vi "GetMotorStatus.vi"() -> (0 "status":T1)   [LabVIEW 2012]
panel:
  in  "簇":T1
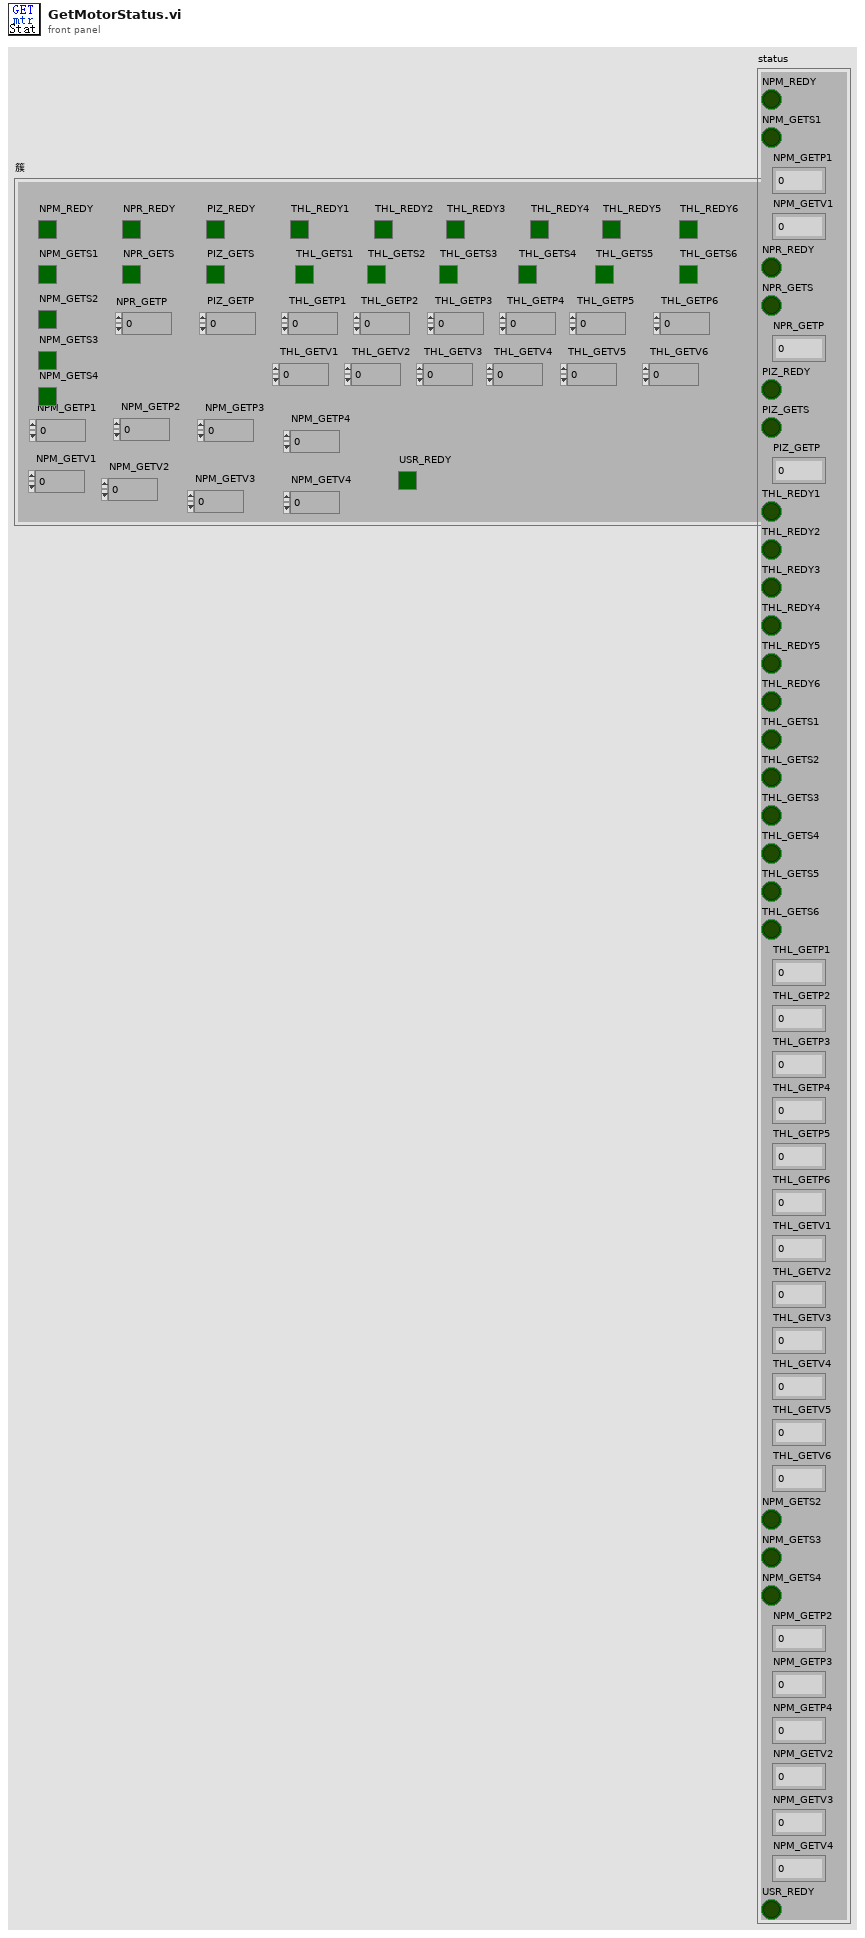
[diagram p1: front panel]
types:
  T1 = cluster{"NPM_REDY":bool, "NPM_GETS1":bool, "NPM_GETP1":dbl, "NPM_GETV1":dbl, "NPR_REDY":bool, "NPR_GETS":bool, "NPR_GETP":dbl, "PIZ_REDY":bool, "PIZ_GETS":bool, "PIZ_GETP":dbl, "THL_REDY1":bool, "THL_REDY2":bool, "THL_REDY3":bool, "THL_REDY4":bool, "THL_REDY5":bool, "THL_REDY6":bool, "THL_GETS1":bool, "THL_GETS2":bool, "THL_GETS3":bool, "THL_GETS4":bool, "THL_GETS5":bool, "THL_GETS6":bool, "THL_GETP1":dbl, "THL_GETP2":dbl, "THL_GETP3":dbl, "THL_GETP4":dbl, "THL_GETP5":dbl, "THL_GETP6":dbl, "THL_GETV1":dbl, "THL_GETV2":dbl, "THL_GETV3":dbl, "THL_GETV4":dbl, "THL_GETV5":dbl, "THL_GETV6":dbl, "NPM_GETS2":bool, "NPM_GETS3":bool, "NPM_GETS4":bool, "NPM_GETP2":dbl, "NPM_GETP3":dbl, "NPM_GETP4":dbl, "NPM_GETV2":dbl, "NPM_GETV3":dbl, "NPM_GETV4":dbl, "USR_REDY":bool}
  T2 = cluster{"DeviceID":string, "Channel":string, "param1":dbl, "Operation":string}
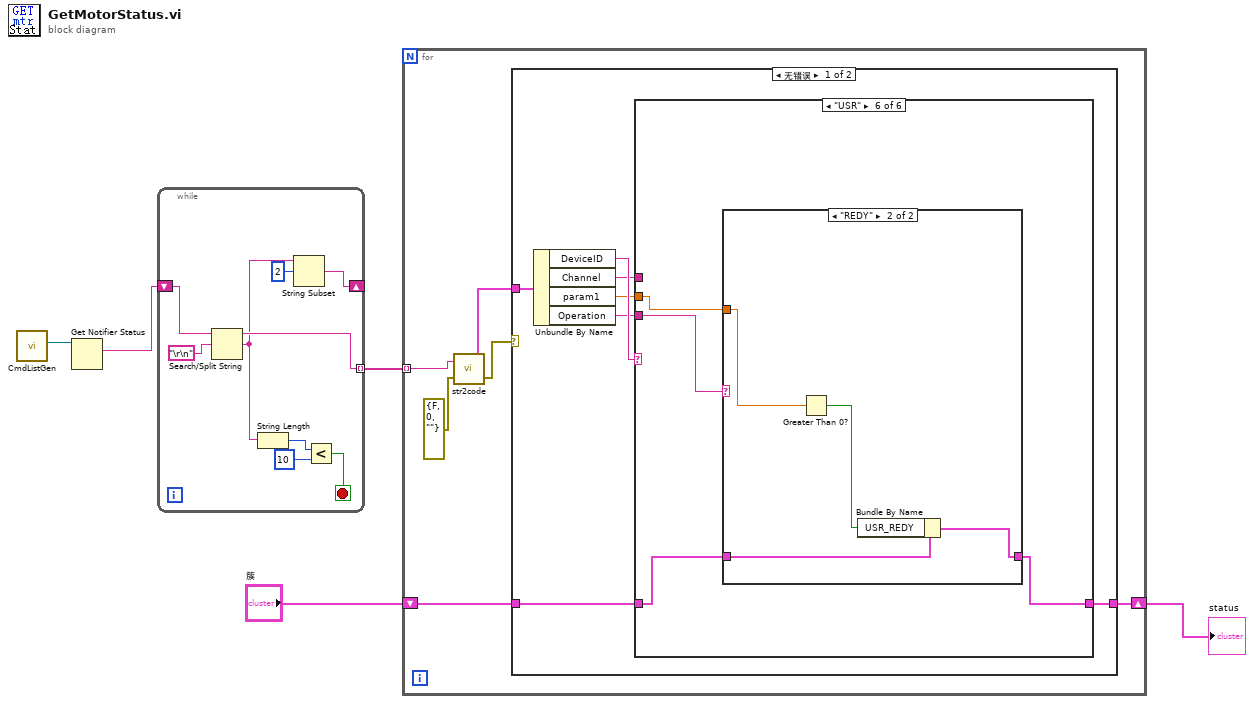
[diagram p0: block diagram]
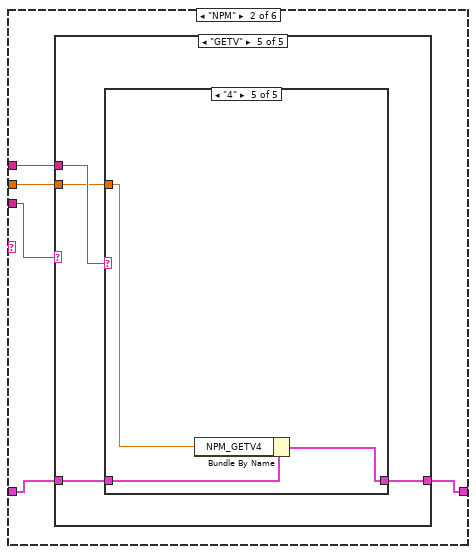
[diagram p3: hidden frame]
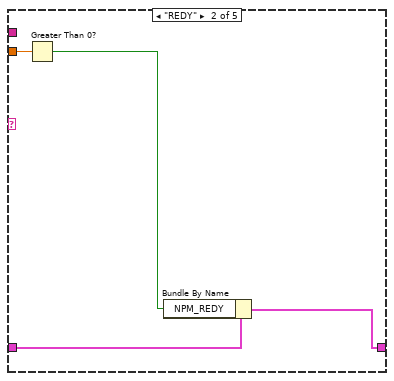
[diagram p5: hidden frame]
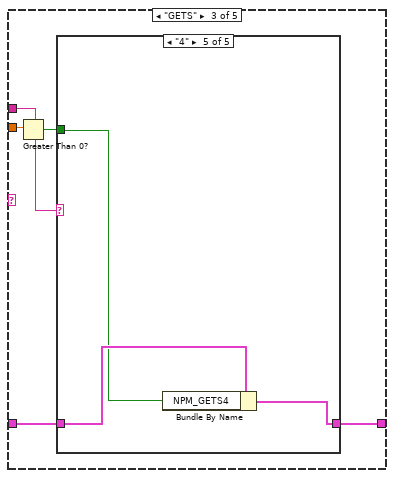
[diagram p6: hidden frame]
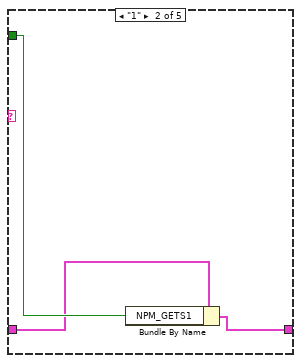
[diagram p8: hidden frame]
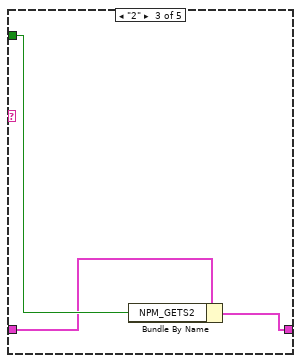
[diagram p9: hidden frame]
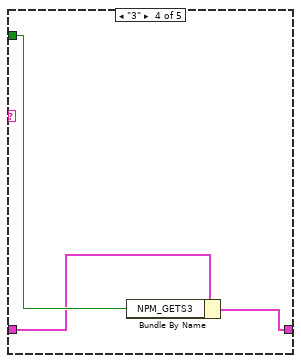
[diagram p10: hidden frame]
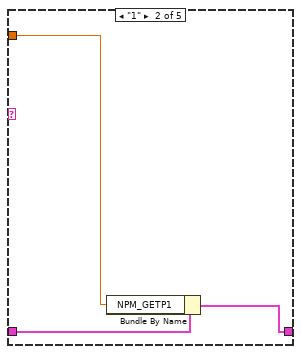
[diagram p12: hidden frame]
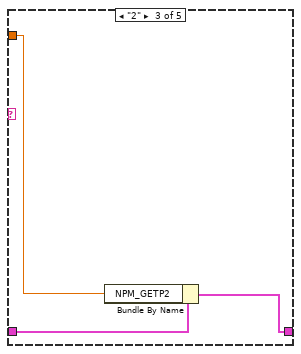
[diagram p13: hidden frame]
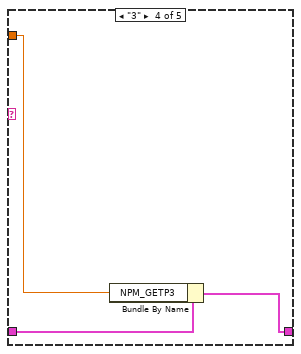
[diagram p14: hidden frame]
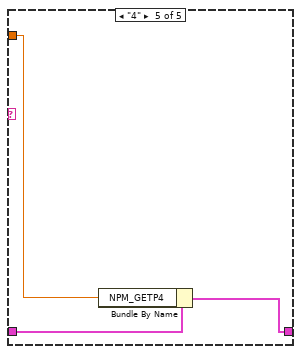
[diagram p15: hidden frame]
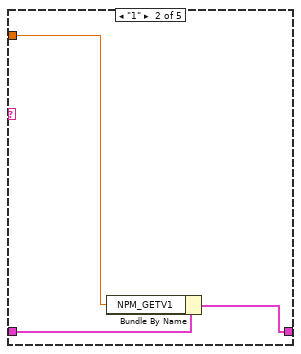
[diagram p17: hidden frame]
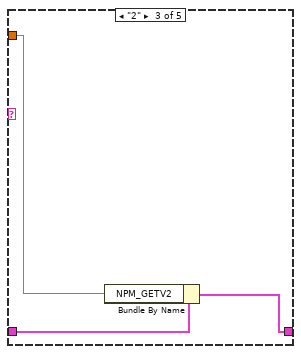
[diagram p18: hidden frame]
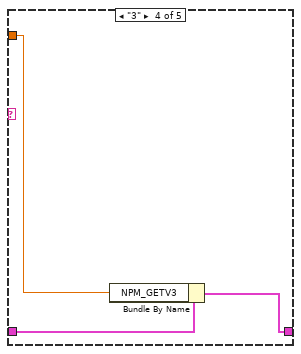
[diagram p19: hidden frame]
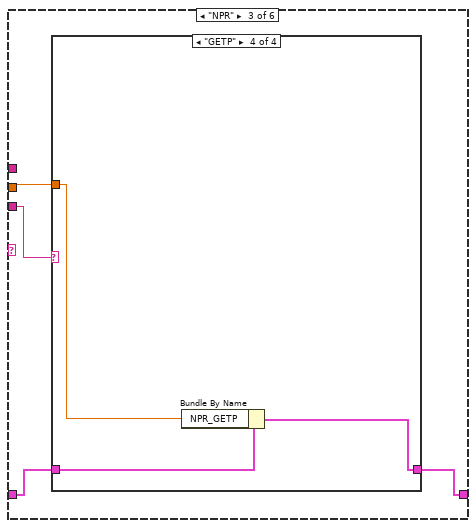
[diagram p20: hidden frame]
diagram:
  n1 = call "CmdListGen.vi"() -> ("StatusNotify"=w3:refnum<notifier>)  [unwired: 1 in, 3 out]
  n2 = Get Notifier Status(notifier=w3) -> (current notification=w5:string)  [unwired: 1 in, 4 out]
  n3 = while {
    shift-right: [w7] -> _
    shift-left: w5 -> [w13]
    tunnel: [w12] -> w4 mode=indexing
    stop <- w9 stop-if-true
    n4 = Search/Split String(string=w13, search string/char (-)="\r\n") -> (substring before match=w12:string, match + rest of string=w8:string)  [unwired: 1 in, 1 out]
    n5 = String Length(string=w8) -> (length=w11:i32)
    n6 = String Subset(string=w8, offset (0)=2 ("偏移量(0)")) -> (substring=w7:string)  [unwired: 1 in]
    n7 = Less?(x=w11, y=10) -> (x < y?=w9:bool)
  }
  n8 = for {
    tunnel: w4 -> [w20] mode=indexing
    shift-right: [w15] -> w1
    shift-left: "簇" -> [w16]
    n9 = call "str2code.vi"("错误输入"=errorcluster {"status"=FALSE, "code"=0, "source"=""}, "input"=w20) -> ("error out"=w18:errorcluster, "Output"=w17:T2)
    n10 = case shown="无错误" w18 {
      tunnel: w17 -> [w27 _]
      tunnel: w16 -> [w22 w232]
      tunnel: [w21 w232] -> w15
      frame No Error {
        n11 = Unbundle By Name(w27) -> ("DeviceID"=w26:string, "Channel"=w25:string, "param1"=w24:dbl, "Operation"=w23:string)
        n12 = case shown="\"USR\"" w26 {
          tunnel: w25 -> [_ w31 _ w109 _ _]
          tunnel: w24 -> [_ w32 w94 w111 w210 w225]
          tunnel: w23 -> [_ w33 w93 w110 w209 w226]
          tunnel: w22 -> [w28 w30 w92 w107 w208 w224]
          tunnel: [w28 w29 w91 w108 w207 w223] -> w21
          frame "", Default {
          }
          frame "NPM" {
            n13 = case shown="\"GETV\"" w33 {
              tunnel: w32 -> [_ w38 w42 w59 w76]
              tunnel: w31 -> [_ _ w43 w60 w77]
              tunnel: w30 -> [w34 w37 w40 w57 w74]
              tunnel: [w34 w36 w39 w58 w75] -> w29
              frame "", Default {
              }
              frame "REDY" {
                n14 = Greater Than 0?(x=w38) -> (x > 0?=w35:bool)
                n15 = Bundle By Name(cluster=w37, "NPM_REDY"=w35) -> (w36:T1)
              }
              frame "GETS" {
                n16 = Greater Than 0?(x=w42) -> (x > 0?=w41:bool)
                n17 = case shown="\"4\"" w43 {
                  tunnel: w41 -> [_ w47 w50 w53 w55]
                  tunnel: w40 -> [w44 w46 w49 w52 w56]
                  tunnel: [w44 w45 w48 w51 w54] -> w39
                  frame "假", Default {
                  }
                  frame "1" {
                    n18 = Bundle By Name(cluster=w46, "NPM_GETS1"=w47) -> (w45:T1)
                  }
                  frame "2" {
                    n19 = Bundle By Name(cluster=w49, "NPM_GETS2"=w50) -> (w48:T1)
                  }
                  frame "3" {
                    n20 = Bundle By Name(cluster=w52, "NPM_GETS3"=w53) -> (w51:T1)
                  }
                  frame "4" {
                    n21 = Bundle By Name(cluster=w56, "NPM_GETS4"=w55) -> (w54:T1)
                  }
                }
              }
              frame "GETP" {
                n22 = case shown="\"假\", 默认" w60 {
                  tunnel: w59 -> [_ w62 w66 w70 w73]
                  tunnel: [w61 w63 w65 w68 w71] -> w58
                  tunnel: w57 -> [w61 w64 w67 w69 w72]
                  frame "假", Default {
                  }
                  frame "1" {
                    n23 = Bundle By Name(cluster=w64, "NPM_GETP1"=w62) -> (w63:T1)
                  }
                  frame "2" {
                    n24 = Bundle By Name(cluster=w67, "NPM_GETP2"=w66) -> (w65:T1)
                  }
                  frame "3" {
                    n25 = Bundle By Name(cluster=w69, "NPM_GETP3"=w70) -> (w68:T1)
                  }
                  frame "4" {
                    n26 = Bundle By Name(cluster=w72, "NPM_GETP4"=w73) -> (w71:T1)
                  }
                }
              }
              frame "GETV" {
                n27 = case shown="\"4\"" w77 {
                  tunnel: w76 -> [_ w79 w83 w87 w90]
                  tunnel: [w78 w80 w82 w85 w88] -> w75
                  tunnel: w74 -> [w78 w81 w84 w86 w89]
                  frame "假", Default {
                  }
                  frame "1" {
                    n28 = Bundle By Name(cluster=w81, "NPM_GETV1"=w79) -> (w80:T1)
                  }
                  frame "2" {
                    n29 = Bundle By Name(cluster=w84, "NPM_GETV2"=w83) -> (w82:T1)
                  }
                  frame "3" {
                    n30 = Bundle By Name(cluster=w86, "NPM_GETV3"=w87) -> (w85:T1)
                  }
                  frame "4" {
                    n31 = Bundle By Name(cluster=w89, "NPM_GETV4"=w90) -> (w88:T1)
                  }
                }
              }
            }
          }
          frame "NPR" {
            n32 = case shown="\"GETP\"" w93 {
              tunnel: w94 -> [_ w99 w103 w105]
              tunnel: w92 -> [w95 w98 w102 w106]
              tunnel: [w95 w96 w101 w104] -> w91
              frame "", Default {
              }
              frame "REDY" {
                n33 = Greater Than 0?(x=w99) -> (x > 0?=w97:bool)
                n34 = Bundle By Name(cluster=w98, "NPR_REDY"=w97) -> (w96:T1)
              }
              frame "GETS" {
                n35 = Greater Than 0?(x=w103) -> (x > 0?=w100:bool)
                n36 = Bundle By Name(cluster=w102, "NPR_GETS"=w100) -> (w101:T1)
              }
              frame "GETP" {
                n37 = Bundle By Name(cluster=w106, "NPR_GETP"=w105) -> (w104:T1)
              }
            }
          }
          frame "THL" {
            n38 = case shown="\"GETV\"" w110 {
              tunnel: w111 -> [_ w117 w141 w163 w186]
              tunnel: w109 -> [_ w115 w139 w164 w187]
              tunnel: [w112 w113 w137 w161 w184] -> w108
              tunnel: w107 -> [w112 w114 w138 w162 w185]
              frame "", Default {
              }
              frame "REDY" {
                n39 = Greater Than 0?(x=w117) -> (x > 0?=w116:bool)
                n40 = case shown="\"6\"" w115 {
                  tunnel: w116 -> [_ w119 w122 w125 w130 w131 w136]
                  tunnel: w114 -> [w118 w121 w124 w127 w129 w133 w135]
                  tunnel: [w118 w120 w123 w126 w128 w132 w134] -> w113
                  frame "", Default {
                  }
                  frame "1" {
                    n41 = Bundle By Name(cluster=w121, "THL_REDY1"=w119) -> (w120:T1)
                  }
                  frame "2" {
                    n42 = Bundle By Name(cluster=w124, "THL_REDY2"=w122) -> (w123:T1)
                  }
                  frame "3" {
                    n43 = Bundle By Name(cluster=w127, "THL_REDY3"=w125) -> (w126:T1)
                  }
                  frame "4" {
                    n44 = Bundle By Name(cluster=w129, "THL_REDY4"=w130) -> (w128:T1)
                  }
                  frame "5" {
                    n45 = Bundle By Name(cluster=w133, "THL_REDY5"=w131) -> (w132:T1)
                  }
                  frame "6" {
                    n46 = Bundle By Name(cluster=w135, "THL_REDY6"=w136) -> (w134:T1)
                  }
                }
              }
              frame "GETS" {
                n47 = Greater Than 0?(x=w141) -> (x > 0?=w140:bool)
                n48 = case shown="\"6\"" w139 {
                  tunnel: w140 -> [_ w145 w148 w151 w154 w155 w158]
                  tunnel: w138 -> [w142 w144 w147 w150 w153 w157 w160]
                  tunnel: [w142 w143 w146 w149 w152 w156 w159] -> w137
                  frame "", Default {
                  }
                  frame "1" {
                    n49 = Bundle By Name(cluster=w144, "THL_GETS1"=w145) -> (w143:T1)
                  }
                  frame "2" {
                    n50 = Bundle By Name(cluster=w147, "THL_GETS2"=w148) -> (w146:T1)
                  }
                  frame "3" {
                    n51 = Bundle By Name(cluster=w150, "THL_GETS3"=w151) -> (w149:T1)
                  }
                  frame "4" {
                    n52 = Bundle By Name(cluster=w153, "THL_GETS4"=w154) -> (w152:T1)
                  }
                  frame "5" {
                    n53 = Bundle By Name(cluster=w157, "THL_GETS5"=w155) -> (w156:T1)
                  }
                  frame "6" {
                    n54 = Bundle By Name(cluster=w160, "THL_GETS6"=w158) -> (w159:T1)
                  }
                }
              }
              frame "GETP" {
                n55 = case shown="\"6\"" w164 {
                  tunnel: w163 -> [_ w166 w169 w172 w175 w178 w181]
                  tunnel: w162 -> [w165 w168 w171 w174 w177 w180 w183]
                  tunnel: [w165 w167 w170 w173 w176 w179 w182] -> w161
                  frame "", Default {
                  }
                  frame "1" {
                    n56 = Bundle By Name(cluster=w168, "THL_GETP1"=w166) -> (w167:T1)
                  }
                  frame "2" {
                    n57 = Bundle By Name(cluster=w171, "THL_GETP2"=w169) -> (w170:T1)
                  }
                  frame "3" {
                    n58 = Bundle By Name(cluster=w174, "THL_GETP3"=w172) -> (w173:T1)
                  }
                  frame "4" {
                    n59 = Bundle By Name(cluster=w177, "THL_GETP4"=w175) -> (w176:T1)
                  }
                  frame "5" {
                    n60 = Bundle By Name(cluster=w180, "THL_GETP5"=w178) -> (w179:T1)
                  }
                  frame "6" {
                    n61 = Bundle By Name(cluster=w183, "THL_GETP6"=w181) -> (w182:T1)
                  }
                }
              }
              frame "GETV" {
                n62 = case shown="\"6\"" w187 {
                  tunnel: w186 -> [_ w189 w192 w195 w198 w201 w204]
                  tunnel: w185 -> [w188 w191 w194 w197 w200 w203 w206]
                  tunnel: [w188 w190 w193 w196 w199 w202 w205] -> w184
                  frame "", Default {
                  }
                  frame "1" {
                    n63 = Bundle By Name(cluster=w191, "THL_GETV1"=w189) -> (w190:T1)
                  }
                  frame "2" {
                    n64 = Bundle By Name(cluster=w194, "THL_GETV2"=w192) -> (w193:T1)
                  }
                  frame "3" {
                    n65 = Bundle By Name(cluster=w197, "THL_GETV3"=w195) -> (w196:T1)
                  }
                  frame "4" {
                    n66 = Bundle By Name(cluster=w200, "THL_GETV4"=w198) -> (w199:T1)
                  }
                  frame "5" {
                    n67 = Bundle By Name(cluster=w203, "THL_GETV5"=w201) -> (w202:T1)
                  }
                  frame "6" {
                    n68 = Bundle By Name(cluster=w206, "THL_GETV6"=w204) -> (w205:T1)
                  }
                }
              }
            }
          }
          frame "PIZ" {
            n69 = case shown="\"\", 默认" w209 {
              tunnel: w210 -> [_ w215 w219 w220]
              tunnel: w208 -> [w211 w214 w218 w222]
              tunnel: [w211 w212 w217 w221] -> w207
              frame "", Default {
              }
              frame "REDY" {
                n70 = Greater Than 0?(x=w215) -> (x > 0?=w213:bool)
                n71 = Bundle By Name(cluster=w214, "PIZ_REDY"=w213) -> (w212:T1)
              }
              frame "GETS" {
                n72 = Greater Than 0?(x=w219) -> (x > 0?=w216:bool)
                n73 = Bundle By Name(cluster=w218, "NPR_GETS"=w216) -> (w217:T1)
              }
              frame "GETP" {
                n74 = Bundle By Name(cluster=w222, "PIZ_GETP"=w220) -> (w221:T1)
              }
            }
          }
          frame "USR" {
            n75 = case shown="\"REDY\"" w226 {
              tunnel: w225 -> [_ w229]
              tunnel: w224 -> [w227 w231]
              tunnel: [w227 w230] -> w223
              frame "\u0000", Default {
              }
              frame "REDY" {
                n76 = Greater Than 0?(x=w229) -> (x > 0?=w228:bool)
                n77 = Bundle By Name(cluster=w231, "USR_REDY"=w228) -> (w230:T1)
              }
            }
          }
        }
      }
      frame Error {
      }
    }
  }
  "status" <- w1
